vi "Auto_Initialization.vi"   [LabVIEW 2011]
uses:
  Auto_Conf.vi
types:
  T1 = typedef "WPI_GyroDevRef.ctl" = cluster{"DevStatus":errorcluster, "Analog Module":T2, "Analog Channel":T3, "Offset":dbl, "Gain (VoltsPerDegree/Second)":dbl}
  T2 = typedef "FPGA_TypedefAnalogModule.ctl" = enum16{"Analog Module 1", "Analog Module 2"}
  T3 = typedef "FPGA_AIChannel.ctl" = enum8{"AI 1", "AI 2", "AI 3", "AI 4", "AI 5", "AI 6", "AI 7", "AI 8", "Invalid"}
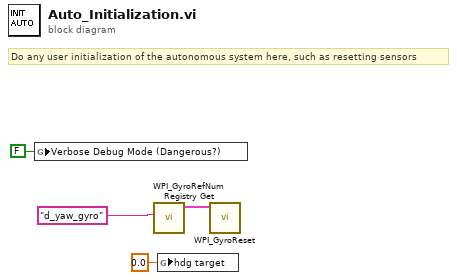
[diagram p0: block diagram]
diagram:
  # "Do any user initialization of the autonomous system here, such as resetting sensors"
  n1 = global write "Auto_Conf.vi" "Verbose Debug Mode (Dangerous?)"(FALSE ("Verbose Debug Mode (Dangerous?)")) -> ()
  n2 = call <vilib>:"WPI_GyroRefNum Registry Get.vi"("refnum name"="d_yaw_gyro") -> ("GyroDevRef"=w4:T1)  [unwired: 1 in, 9 out]
  n3 = global write "Auto_Conf.vi" "hdg target"(0.0 ("hdg target")) -> ()
  n4 = call <vilib>:"WPI_GyroReset.vi"("GyroDevRef"=w4) -> ()  [unwired: 11 out]
